vi "ConvertPayloadStrToPayload.vi"(11 "CAN Data":string="55 55 05 00 00 00 00 00") -> (3 "payload":u8[](array[numeric]) format="%x")   [LabVIEW 2018, in "Library-DataConvert.lvlib"]
uses:
  Library-DataConvert.lvlib
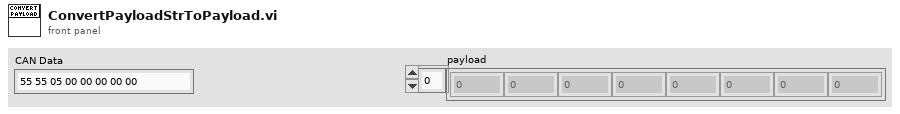
[diagram p1: front panel]
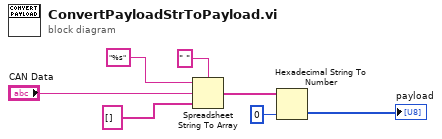
[diagram p0: block diagram]
diagram:
  n1 = Spreadsheet String To Array(delimiter (Tab)=" " ("구분 문자(탭)"), format string="%s" ("포맷 문자열"), spreadsheet string="CAN Data", array type (2D Dbl)=string[] []) -> (array=w7:string[])
  n2 = Hexadecimal String To Number(string=w7, default (0uL)=u8 0 ("기본(0 U32)")) -> (number=→"payload":u8[])  [unwired: 1 in, 1 out]
